vi "Set_Control_State.vi"(8 "Status/Errors in":refnum<vi>, 9 "Control Parameters [] in":T15[](array[typedef]) {"Aux Byte Value" format="%02x"; "Max Real Value" format="%#_6e"; "Min Real Value" format="%#_6e"; "dReal/dByte" format="%#_6e"; "Byte Value" format="%02x"; "Identifier" format="%02x"}, 10 "Main parameters in":T1={"Mode"={"Mode"=enum."Dialog", "Expert?"=FALSE, "Dialog?"=FALSE}, "Stop loop"={"Settings changed?"=FALSE, "Stop?"=refnum}, "Send message"={"Send mode"=enum."Get parameters", "Set parameter list"=0, "Get parameter list"=0, "Reset device"=0, "Length set settings message"=0, "Reset buttons?"=FALSE, "Reset Master?"=enum."General"}, "Write settings"={"Options"=enum."File 1"}, "Settings state"={"MAS locked?"=refnum, "SLV locked?"=refnum}, "Button refs"={"Stop program"=refnum, "Save settings"=refnum, "DAQ mode"=refnum, "Reset settings"=refnum, "Apply settings"=refnum, "Reset MAS"=refnum, "Reset SLV"=refnum, "Local DBase?"=refnum, "Last value DBase"=FALSE, "Database"=refnum, "Calibration"=refnum, "Save settings 2"=refnum}, "Update screen"={"Detector number"=0, "Hardware"=enum."None"}, "Files"={"Path config file"=path "", "Path def. ini file"=path "", "Path ini file 1"=path "", "Path ini file 2"=path "", "Path RBF file"=path ""}, "DB connection"={"connection reference"=refnum, "Connected?"=refnum, "ODBC Name"=""}, "Status_id"=refnum, "Time difference"=refnum, "Satellites"=refnum, "Alignment parameters"=refnum, "Page Statistics 2"=refnum, "Database"=refnum, "Page Statistics"=refnum} {"Update screen"."Detector number" format="%#.0f"; "Send message"."Reset device" format="%x"; "Send message"."Get parameter list" format="%x"; "Send message"."Set parameter list" format="%x"}) -> (0 "Status/Errors out":refnum<vi>, 1 "Control Parameters [] out":T15[](array[typedef]) {"Aux Byte Value" format="%02x"; "Max Real Value" format="%#_6e"; "Min Real Value" format="%#_6e"; "dReal/dByte" format="%#_6e"; "Byte Value" format="%02x"; "Identifier" format="%02x"}, 2 "Main parameters out":T1={"Mode"={"Mode"=enum."Dialog", "Expert?"=FALSE, "Dialog?"=FALSE}, "Stop loop"={"Settings changed?"=FALSE, "Stop?"=refnum}, "Send message"={"Send mode"=enum."Get parameters", "Set parameter list"=0, "Get parameter list"=0, "Reset device"=0, "Length set settings message"=0, "Reset buttons?"=FALSE, "Reset Master?"=enum."General"}, "Write settings"={"Options"=enum."File 1"}, "Settings state"={"MAS locked?"=refnum, "SLV locked?"=refnum}, "Button refs"={"Stop program"=refnum, "Save settings"=refnum, "DAQ mode"=refnum, "Reset settings"=refnum, "Apply settings"=refnum, "Reset MAS"=refnum, "Reset SLV"=refnum, "Local DBase?"=refnum, "Last value DBase"=FALSE, "Database"=refnum, "Calibration"=refnum, "Save settings 2"=refnum}, "Update screen"={"Detector number"=0, "Hardware"=enum."None"}, "Files"={"Path config file"=path "", "Path def. ini file"=path "", "Path ini file 1"=path "", "Path ini file 2"=path "", "Path RBF file"=path ""}, "DB connection"={"connection reference"=refnum, "Connected?"=refnum, "ODBC Name"=""}, "Status_id"=refnum, "Time difference"=refnum, "Satellites"=refnum, "Alignment parameters"=refnum, "Page Statistics 2"=refnum, "Database"=refnum, "Page Statistics"=refnum} {"Update screen"."Detector number" format="%#.0f"; "Send message"."Reset device" format="%x"; "Send message"."Get parameter list" format="%x"; "Send message"."Set parameter list" format="%x"})   [LabVIEW 2013]
uses:
  Controls/Control_Parameters.ctl
  Controls/Master.ctl
  Controls/Main_Parameters.ctl
  Controls/Mode.ctl
  Controls/Stop_Loop.ctl
  Controls/Send_Message.ctl
  Controls/Send_Message_Mode.ctl
  Controls/Write_Settings.ctl
  Controls/Write_Settings_Options.ctl
  Controls/Settings_State.ctl
  Controls/Button_Refs.ctl
  Controls/Update_Screen.ctl
  Controls/Files.ctl
  Controls/DB_Connection.ctl
  database/Connection.llb/Conn ObjectReference.ctl
  Controls/Get_Set_Buttons_mode.ctl
  Controls/TabPage_Events.ctl
  Controls/TabPage_Statistics.ctl
  Controls/Page_Thresholds.ctl
  Controls/Get_Set_Statistics_Options.ctl
  Controls/TabPage_Statistics2.ctl
  Controls/Tabpage_Satellites.ctl
panel:
  out "Last trigger Stack":u64[](array[numeric])
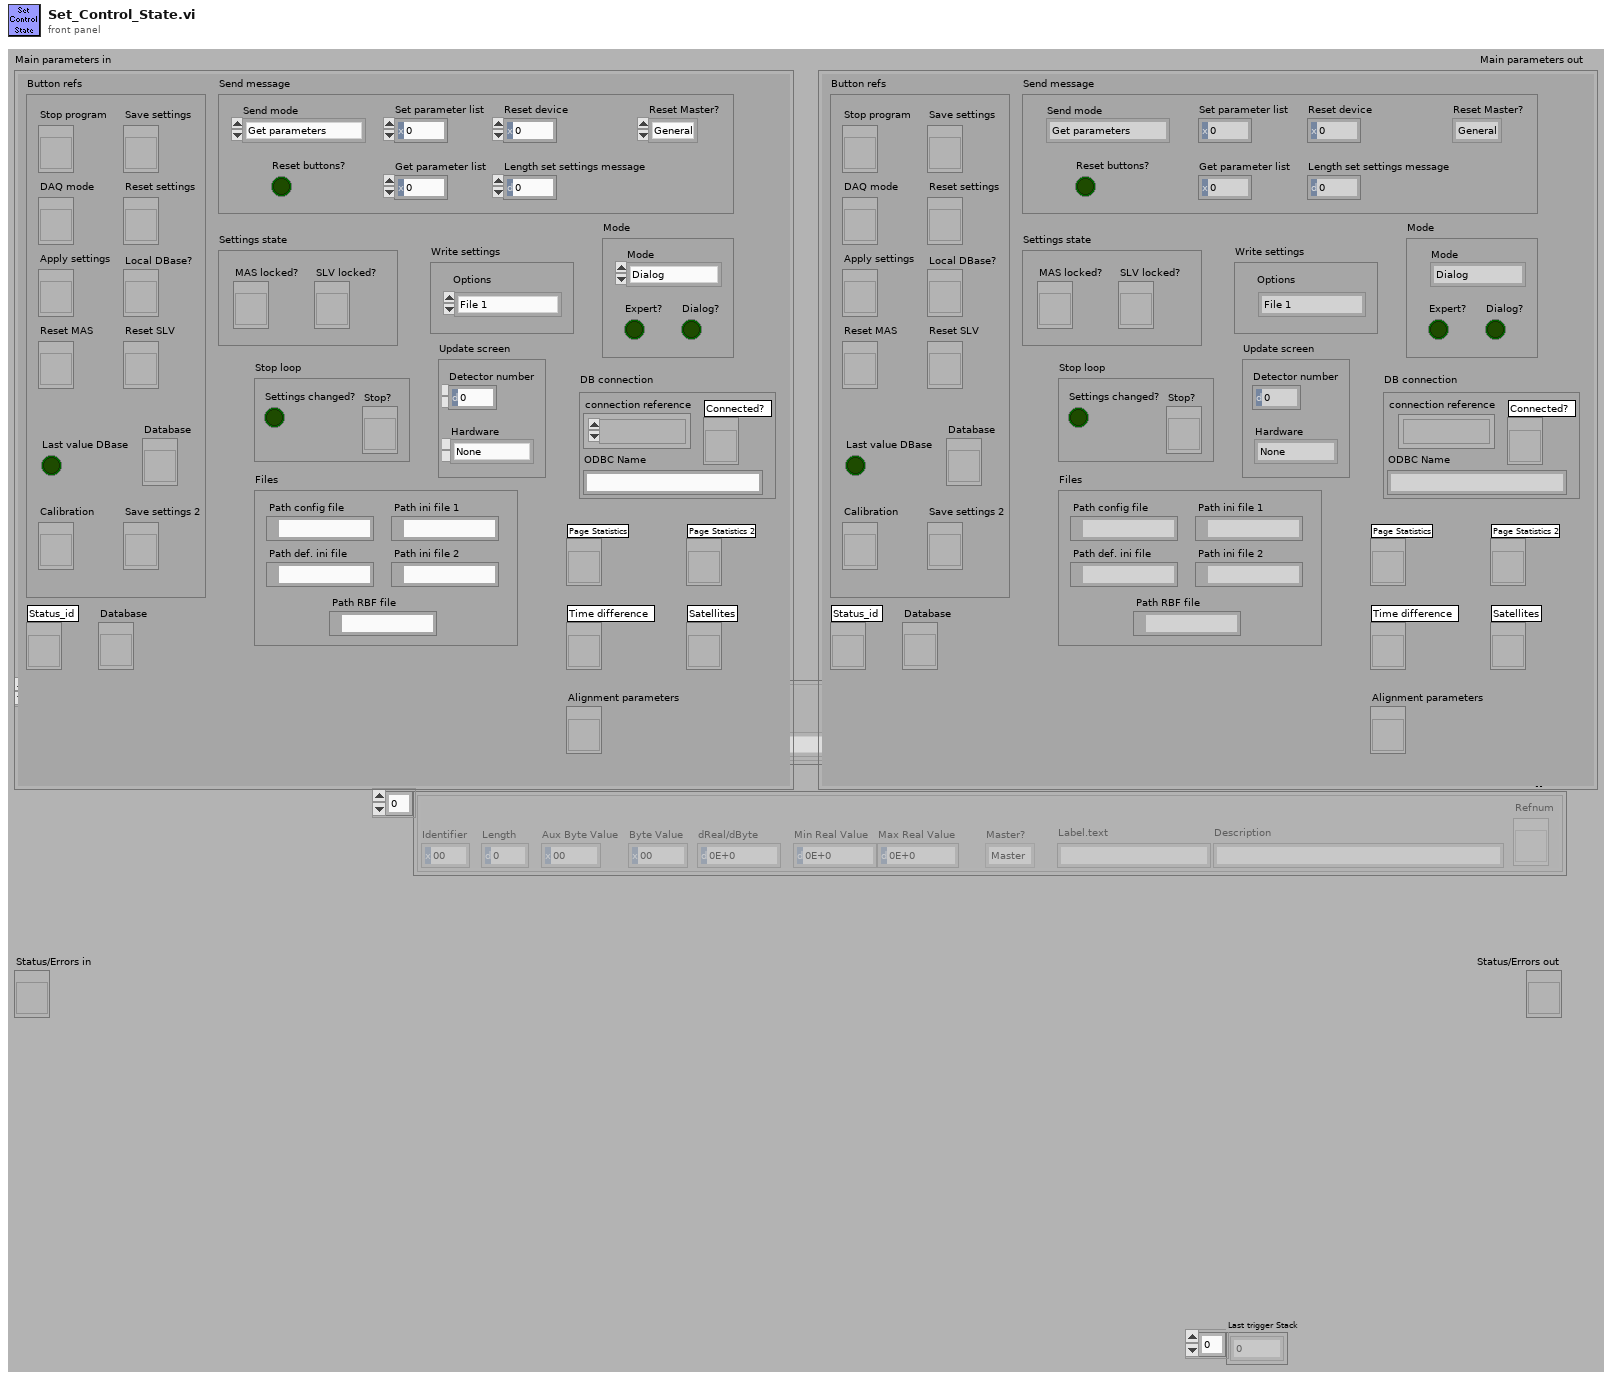
[diagram p1: front panel]
types:
  T1 = typedef "Main_Parameters.ctl" = cluster{"Mode":T2, "Stop loop":T3, "Send message":T4, "Write settings":T7, "Settings state":T9, "Button refs":T10, "Update screen":T11, "Files":T12, "DB connection":T13, "Status_id":refnum<vi>, "Time difference":refnum<vi>, "Satellites":refnum<vi>, "Alignment parameters":refnum<vi>, "Page Statistics 2":refnum<vi>, "Database":refnum<vi>, "Page Statistics":refnum<vi>}
  T2 = typedef "Mode.ctl" = cluster{"Mode":enum8{"Stop", "Dialog", "Hisparc II", "Hisparc II DAQ", "Alignment"}, "Expert?":bool, "Dialog?":bool}
  T3 = typedef "Stop_Loop.ctl" = cluster{"Settings changed?":bool, "Stop?":refnum<vi>}
  T4 = typedef "Send_Message.ctl" = cluster{"Send mode":T5, "Set parameter list":u8, "Get parameter list":u8, "Reset device":u8, "Length set settings message":i32, "Reset buttons?":bool, "Reset Master?":T6}
  T5 = typedef "Send_Message_Mode.ctl" = enum16{"Get parameters", "Set parameters", "From front panel", "From parameters", "Reset device", "Alignment"}
  T6 = typedef "Master.ctl" = enum16{"Master", "Slave", "General"}
  T7 = typedef "Write_Settings.ctl" = cluster{"Options":T8}
  T8 = typedef "Write_Settings_Options.ctl" = enum16{"File 1", "File 2", "Alignment", "Reset"}
  T9 = typedef "Settings_State.ctl" = cluster{"MAS locked?":refnum<vi>, "SLV locked?":refnum<vi>}
  T10 = typedef "Button_Refs.ctl" = cluster{"Stop program":refnum<vi>, "Save settings":refnum<vi>, "DAQ mode":refnum<vi>, "Reset settings":refnum<vi>, "Apply settings":refnum<vi>, "Reset MAS":refnum<vi>, "Reset SLV":refnum<vi>, "Local DBase?":refnum<vi>, "Last value DBase":bool, "Database":refnum<vi>, "Calibration":refnum<vi>, "Save settings 2":refnum<vi>}
  T11 = typedef "Update_Screen.ctl" = cluster{"Detector number":u16, "Hardware":enum8{"None", "HiSPARC I", "HiSPARC II", "HiSPARC III", "Unknown"}}
  T12 = typedef "Files.ctl" = cluster{"Path config file":path, "Path def. ini file":path, "Path ini file 1":path, "Path ini file 2":path, "Path RBF file":path}
  T13 = typedef "DB_Connection.ctl" = cluster{"connection reference":T14, "Connected?":refnum<vi>, "ODBC Name":string}
  T14 = typedef "Conn ObjectReference.ctl" = refnum<k1>
  T15 = typedef "Control_Parameters.ctl" = cluster{"Identifier":u8, "Length":u16, "Byte Value":u32, "dReal/dByte":dbl, "Min Real Value":dbl, "Max Real Value":dbl, "Master?":T6, "Label.text":string, "Description":string, "Refnum":refnum<vi>, "Aux Byte Value":u32}
  T16 = typedef "Tabpage_Satellites.ctl" = cluster{"Satellites_online":dbl[], "Satellite_signal":dbl[][], "Total_signal_strength":dbl[], "First time?":bool}
  T17 = typedef "TabPage_Statistics2.ctl" = cluster{"Baseline_overshoot":dbl, "St.Dev.overshoot":dbl, "Data points overshoot":dbl, "Time difference overshoot":dbl, "Time_difference_zoom_count":dbl, "Baseline.His":cluster{"t0":i32, "dt":i32, "Histogram":i32[][]}, "St._dev.His":cluster{"t0":i32, "dt":i32, "Histogram":i32[][]}, "Trace_length.His":cluster{"t0":i32, "dt":i32, "Histogram":i32[][]}, "Time_difference.His_zoom":cluster{"t0":i32, "dt":i32, "Histogram":i32[][]}, "Time_difference.His":cluster{"t0":i32, "dt":i32, "Histogram":i32[][]}, "Baselin Entries":u64, "Baseline Overshoots":u64, "Time Entries ":u64, "Time  Overshoots ":u64, "St.dev. Entries ":u64, "St.dev.  Overshoots ":u64, "Length  Entries ":u64, "Length Overshoots ":u64, "Time zoom Entries ":u64, "Time zoom Overshoots ":u64}
  T18 = typedef "Get_Set_Statistics_Options.ctl" = enum16{"Get", "Set singles", "Set events"}
  T19 = typedef "TabPage_Statistics.ctl" = cluster{"Thresh_Count_MAS":T20, "Thresh_Count_SLV":T20, "Count":bool, "Time_to_count":u32, "Time":u32, "Time_to_count_ref":refnum<vi>, "Counting?":bool, "Baseline_MAS_Ch1":i16, "Baseline_MAS_Ch2":i16, "Baseline_SLV_Ch1":i16, "Baseline_SLV_Ch2":i16, "Basel_Err_MAS_Ch1":u32, "Basel_Err_MAS_Ch2":u32, "Basel_Err_SLV_Ch1":u32, "Basel_Err_SLV_Ch2":u32, "Peaks_Overshoot":dbl, "Height_Overshoot":dbl, "Integrals_Overshoot":dbl, "Last_event":dbl, "Total_Trigger":u32, "Av_Trigger":dbl, "Number of peaks":cluster{"t0":i32, "dt":i32, "Histogram":i32[][]}, "Pulse height":cluster{"t0":i32, "dt":i32, "Histogram":i32[][]}, "Integral":cluster{"t0":i32, "dt":i32, "Histogram":i32[][]}, "Number of peaks Entries":u64, "Number of peaks Overshoots":u64, "Pulse height  Entries":u64, "Pulse height Overshoots":u64, "Integral Entries":u64, "Integral Overshoots":u64, "Last trigger Stack":refnum<vi>}
  T20 = typedef "Page_Thresholds.ctl" = cluster{"Sing_Ch1_low":u32, "Sing_Ch1_high":u32, "Sing_Ch2_low":u32, "Sing_Ch2_high":u32, "Total_Ch1_low":u32, "Total_Ch1_high":u32, "Total_Ch2_low":u32, "Total_Ch2_high":u32, "Av_Ch1_low":dbl, "Av_Ch1_high":dbl, "Av_Ch2_low":dbl, "Av_Ch2_high":dbl}
  T21 = typedef "TabPage_Events.ctl" = cluster{"Det_Numb":u16, "GPS_Timestamp":string, "Trigger_Pattern":cluster{"Master ch. 1 lower threshold":bool, "Master ch. 1 higher threshold":bool, "Master ch. 2 lower threshold":bool, "Master ch. 2 higher threshold":bool, "Slave ch. 1 lower threshold":bool, "Slave ch. 1 higher threshold":bool, "Slave ch. 2 lower threshold":bool, "Slave ch. 2 higher threshold":bool, "External trigger":bool, "Slave present?":bool, "Ch. 1 low comparator master":bool, "Ch. 1 high comparator master":bool, "Ch. 2 low comparator master":bool, "Ch. 2 high comparator master":bool, "Ch. 1 low comparator slave":bool, "Ch. 1 high comparator slave":bool, "Ch. 2 low comparator slave":bool, "Ch. 2 high comparator slave":bool}, "Traces":dbl[][], "MAS_Status_Events":bool, "MAS_Vers_Numb":string, "SLV_Status_Events":bool, "SLV_Vers_Numb":string, "DBase_connected?":bool, "MAS_GPS_Long":dbl, "MAS_GPS_Lat":dbl, "MAS_GPS_Alt":dbl, "Hardware":enum8{"None", "HiSPARC I", "HiSPARC II", "HiSPARC III", "Unknown"}}
  T22 = typedef "Get_Set_Buttons_mode.ctl" = enum16{"Get", "Get DAQ", "Set", "Set settings"}
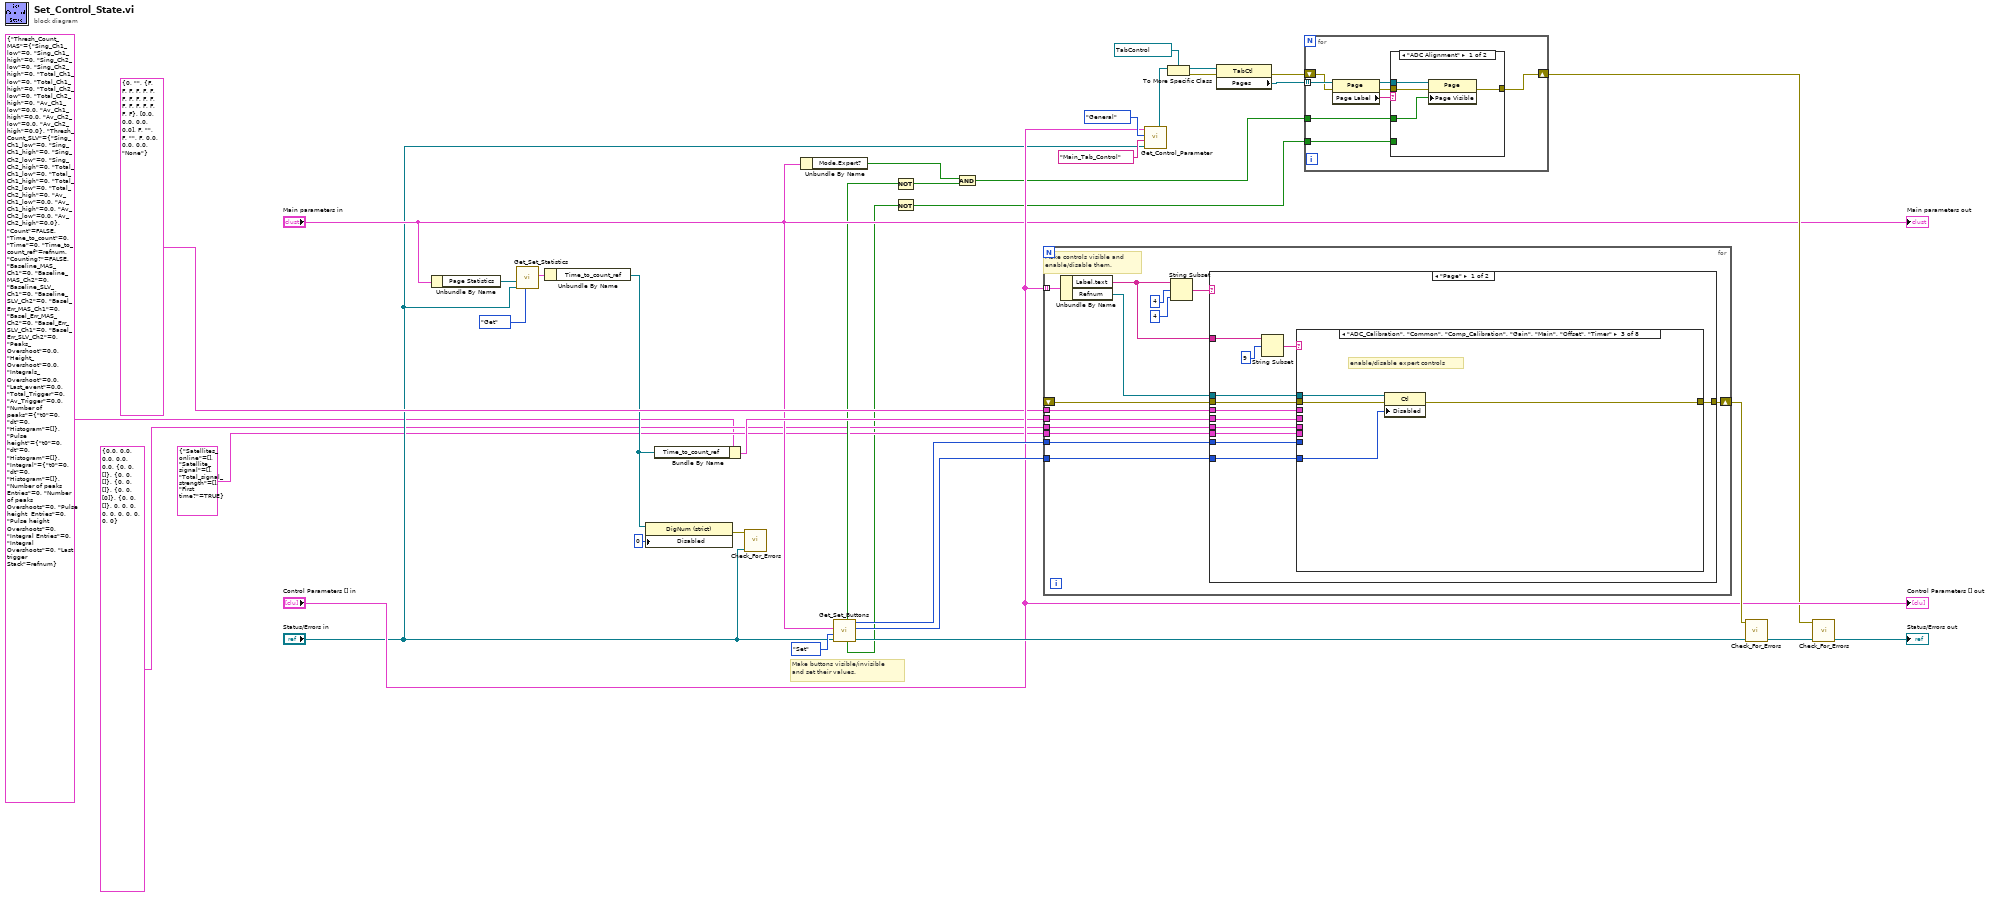
[diagram p0: block diagram]
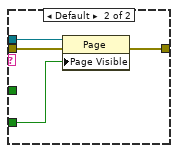
[diagram p2: hidden frame]
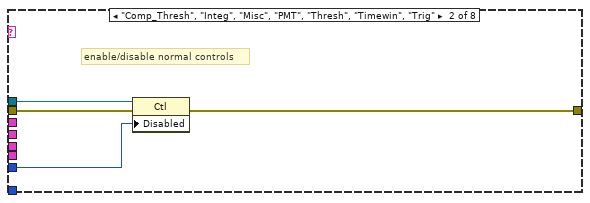
[diagram p4: hidden frame]
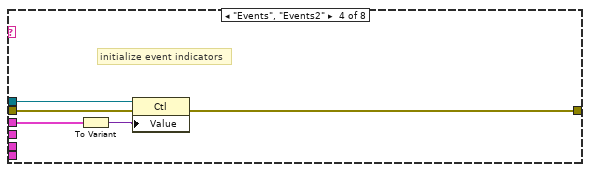
[diagram p5: hidden frame]
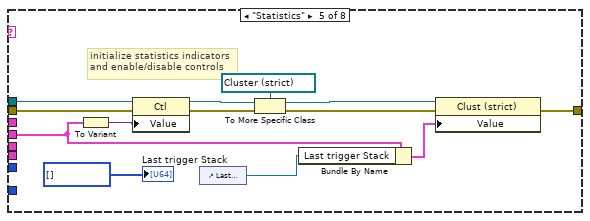
[diagram p6: hidden frame]
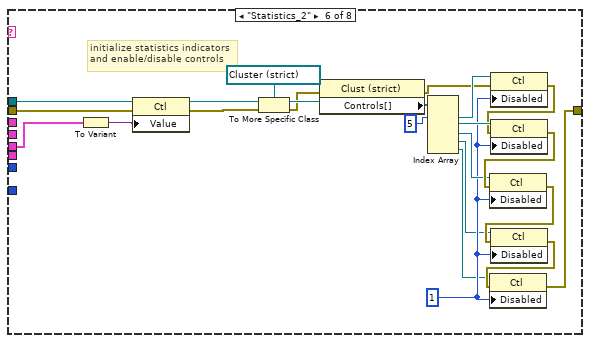
[diagram p7: hidden frame]
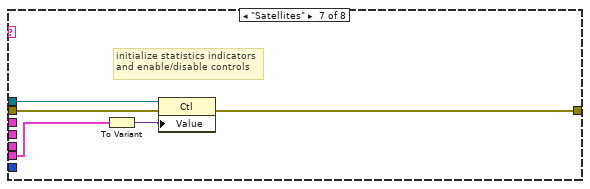
[diagram p8: hidden frame]
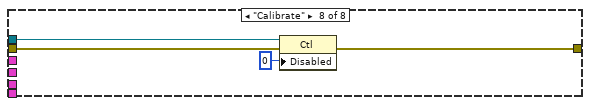
[diagram p9: hidden frame]
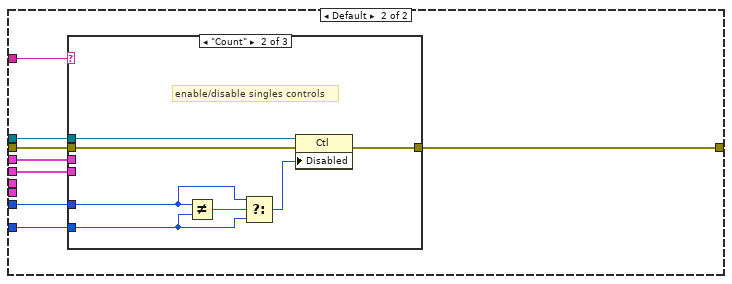
[diagram p10: hidden frame]
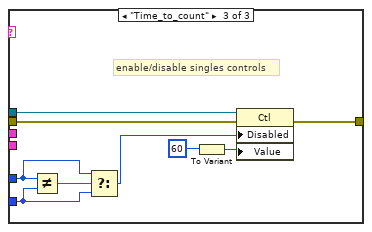
[diagram p12: hidden frame]
diagram:
  # "Make buttons visible/invisible\nand set their values."
  # "Make controls visible and\nenable/disable them."
  n1 = Unbundle By Name("Main parameters in") -> ("Page Statistics"=w1:refnum<vi>)
  n2 = call "Get_Set_Statistics.vi"("Page Statistics in"=w1, "Status/Errors in"="Status/Errors in", "Get/Set"=Get_Set_Statistics_Options."Get") -> ("Value out"=w16:T19)  [unwired: 2 in, 5 out]
  n3 = Unbundle By Name(w16) -> ("Time_to_count_ref"=w7:refnum<vi>)
  n4 = property class="DigNum (strict)"(reference=w7, "Disabled"=u8 0) -> (error out=w9:errorcluster)  [unwired: 1 in, 1 out]
  n5 = Bundle By Name(cluster=T19 {"Thresh_Count_MAS"={"Sing_Ch1_low"=0, "Sing_Ch1_high"=0, "Sing_Ch2_low"=0, "Sing_Ch2_high"=0, "Total_Ch1_low"=0, "Total_Ch1_high"=0, "Total_Ch2_low"=0, "Total_Ch2_high"=0, "Av_Ch1_low"=0.0, "Av_Ch1_high"=0.0, "Av_Ch2_low"=0.0, "Av_Ch2_high"=0.0}, "Thresh_Count_SLV"={"Sing_Ch1_low"=0, "Sing_Ch1_high"=0, "Sing_Ch2_low"=0, "Sing_Ch2_high"=0, "Total_Ch1_low"=0, "Total_Ch1_high"=0, "Total_Ch2_low"=0, "Total_Ch2_high"=0, "Av_Ch1_low"=0.0, "Av_Ch1_high"=0.0, "Av_Ch2_low"=0.0, "Av_Ch2_high"=0.0}, "Count"=FALSE, "Time_to_count"=0, "Time"=0, "Time_to_count_ref"=refnum, "Counting?"=FALSE, "Baseline_MAS_Ch1"=0, "Baseline_MAS_Ch2"=0, "Baseline_SLV_Ch1"=0, "Baseline_SLV_Ch2"=0, "Basel_Err_MAS_Ch1"=0, "Basel_Err_MAS_Ch2"=0, "Basel_Err_SLV_Ch1"=0, "Basel_Err_SLV_Ch2"=0, "Peaks_Overshoot"=0.0, "Height_Overshoot"=0.0, "Integrals_Overshoot"=0.0, "Last_event"=0.0, "Total_Trigger"=0, "Av_Trigger"=0.0, "Number of peaks"={"t0"=0, "dt"=0, "Histogram"=[]}, "Pulse height"={"t0"=0, "dt"=0, "Histogram"=[]}, "Integral"={"t0"=0, "dt"=0, "Histogram"=[]}, "Number of peaks Entries"=0, "Number of peaks Overshoots"=0, "Pulse height  Entries"=0, "Pulse height Overshoots"=0, "Integral Entries"=0, "Integral Overshoots"=0, "Last trigger Stack"=refnum} ("GEN_Page_Statistics"), "Time_to_count_ref"=w7) -> (w15:T19)
  n6 = call "Check_For_Errors.vi"("Status/Errors in"="Status/Errors in", "error in"=w9) -> ()  [unwired: 10 out]
  n7 = Unbundle By Name("Main parameters in") -> ("Mode.Expert?"=w11:bool)
  n8 = call "Get_Set_Buttons.vi"("Status/Errors in"="Status/Errors in", "Set?"=Get_Set_Buttons_mode."Set", "Main parameters"="Main parameters in") -> ("Status/Errors out"=w32:refnum<vi>, "Enabled State Expert"=w33:u8, "Enabled State Normal"=w34:u8, "Calibration value"=w2:bool, "DAQ mode value"=w13:bool)  [unwired: 1 in, 3 out]
  n9 = Not(x=w13) -> (.not. x?=w12:bool)
  n10 = Not(x=w2) -> (.not. x?=w19:bool)
  n11 = And(x=w11, y=w12) -> (x .and. y?=w10:bool)
  n12 = for {
    tunnel: "Control Parameters [] in" -> [w47] mode=indexing
    tunnel: w34 -> [w45]
    shift-right: [w43] -> w36
    shift-left: _ -> [w44]
    tunnel: w33 -> [w42]
    tunnel: T21 {"Det_Numb"=0, "GPS_Timestamp"="", "Trigger_Pattern"={"Master ch. 1 lower threshold"=FALSE, "Master ch. 1 higher threshold"=FALSE, "Master ch. 2 lower threshold"=FALSE, "Master ch. 2 higher threshold"=FALSE, "Slave ch. 1 lower threshold"=FALSE, "Slave ch. 1 higher threshold"=FALSE, "Slave ch. 2 lower threshold"=FALSE, "Slave ch. 2 higher threshold"=FALSE, "External trigger"=FALSE, "Slave present?"=FALSE, "Ch. 1 low comparator master"=FALSE, "Ch. 1 high comparator master"=FALSE, "Ch. 2 low comparator master"=FALSE, "Ch. 2 high comparator master"=FALSE, "Ch. 1 low comparator slave"=FALSE, "Ch. 1 high comparator slave"=FALSE, "Ch. 2 low comparator slave"=FALSE, "Ch. 2 high comparator slave"=FALSE}, "Traces"=[[0.0, 0.0], [0.0, 0.0]], "MAS_Status_Events"=FALSE, "MAS_Vers_Numb"="", "SLV_Status_Events"=FALSE, "SLV_Vers_Numb"="", "DBase_connected?"=FALSE, "MAS_GPS_Long"=0.0, "MAS_GPS_Lat"=0.0, "MAS_GPS_Alt"=0.0, "Hardware"=enum."None"} ("Events") -> [w40]
    tunnel: w15 -> [w39]
    tunnel: T17 {"Baseline_overshoot"=0.0, "St.Dev.overshoot"=0.0, "Data points overshoot"=0.0, "Time difference overshoot"=0.0, "Time_difference_zoom_count"=0.0, "Baseline.His"={"t0"=0, "dt"=0, "Histogram"=[]}, "St._dev.His"={"t0"=0, "dt"=0, "Histogram"=[]}, "Trace_length.His"={"t0"=0, "dt"=0, "Histogram"=[]}, "Time_difference.His_zoom"={"t0"=0, "dt"=0, "Histogram"=[[0]]}, "Time_difference.His"={"t0"=0, "dt"=0, "Histogram"=[]}, "Baselin Entries"=0, "Baseline Overshoots"=0, "Time Entries "=0, "Time  Overshoots "=0, "St.dev. Entries "=0, "St.dev.  Overshoots "=0, "Length  Entries "=0, "Length Overshoots "=0, "Time zoom Entries "=0, "Time zoom Overshoots "=0} ("GEN_Page_Statistics_2") -> [w38]
    tunnel: T16 {"Satellites_online"=[], "Satellite_signal"=[], "Total_signal_strength"=[], "First time?"=TRUE} ("GEN_Page_Statistics_2") -> [w37]
    n13 = Unbundle By Name(w47) -> ("Label.text"=w46:string, "Refnum"=w41:refnum<vi>)
    n14 = String Subset(string=w46, offset (0)=4, length (rest)=4 ("length (rest)")) -> (substring=w49:string)
    n15 = case shown="\"Page\"" w49 {
      tunnel: w41 -> [w56 w126]
      tunnel: w46 -> [w60 w122]
      tunnel: w45 -> [w59 w129]
      tunnel: w44 -> [w55 w125]
      tunnel: [w58 w128] -> w43
      tunnel: w42 -> [w57 w127]
      tunnel: w40 -> [w54 w124]
      tunnel: w39 -> [w53 w123]
      tunnel: w38 -> [w52 _]
      tunnel: w37 -> [w51 _]
      frame "Page" {
        n16 = String Subset(string=w60, offset (0)=9) -> (substring=w61:string)  [unwired: 1 out]
        n17 = case shown="\"ADC_Calibration\", \"Common\", \"Comp_Calibration\", \"Gain\", \"Main\", \"Offset\", \"Timer\"" w61 {
          tunnel: w56 -> [_ w67 w71 w76 w89 w108 w116 w120]
          tunnel: w59 -> [_ w66 _ _ _ _ _ _]
          tunnel: w55 -> [w63 w65 w70 w75 w88 w112 w115 w119]
          tunnel: [w63 w64 w69 w74 w82 w90 w113 w121] -> w58
          tunnel: w57 -> [_ _ w68 _ _ _ _ _]
          tunnel: w54 -> [_ _ _ w72 _ _ _ _]
          tunnel: w53 -> [_ _ _ _ w79 _ _ _]
          tunnel: w52 -> [_ _ _ _ _ w110 _ _]
          tunnel: w51 -> [_ _ _ _ _ _ w114 _]
          frame Default {
          }
          frame "Comp_Thresh", "Integ", "Misc", "PMT", "Thresh", "Timewin", "Trig" {
            # "enable/disable normal controls"
            n18 = property class="Ctl"(reference=w67, error in=w65, "Disabled"=w66) -> (error out=w64:errorcluster)  [unwired: 1 out]
          }
          frame "ADC_Calibration", "Common", "Comp_Calibration", "Gain", "Main", "Offset", "Timer" {
            # "enable/disable expert controls"
            n19 = property class="Ctl"(reference=w71, error in=w70, "Disabled"=w68) -> (error out=w69:errorcluster)  [unwired: 1 out]
          }
          frame "Events", "Events2" {
            # "initialize event indicators"
            n20 = To Variant(anything=w72) -> (Variant=w73:variant)
            n21 = property class="Ctl"(reference=w76, error in=w75, "Value"=w73) -> (error out=w74:errorcluster)  [unwired: 1 out]
          }
          frame "Statistics" {
            # "initialize statistics indicators\nand enable/disable controls"
            n22 = To Variant(anything=w79) -> (Variant=w87:variant)
            n23 = property class="Ctl"(reference=w89, error in=w88, "Value"=w87) -> (reference out=w84:refnum<vi>, error out=w83:errorcluster)
            n24 = control-ref of="Last trigger Stack"() -> (w81:refnum<vi>)
            n25 = To More Specific Class(target class=refnum<vi> refnum ("GEN_Page_Statistics"), reference=w84, error in=w83) -> (specific class reference=w86:refnum<vi>, error out=w85:errorcluster)
            n26 = Bundle By Name(cluster=w79, "Last trigger Stack"=w81) -> (w78:T19)
            n27 = property class="Clust (strict)"(reference=w86, error in=w85, "Value"=w78) -> (error out=w82:errorcluster)  [unwired: 1 out]
            "Last trigger Stack" <- u64[] [] ("Last trigger Stack")
          }
          frame "Statistics_2" {
            w93 = u8 1 ("index")
            # "initialize statistics indicators\nand enable/disable controls"
            n28 = To Variant(anything=w110) -> (Variant=w111:variant)
            n29 = property class="Ctl"(reference=w108, error in=w112, "Value"=w111) -> (reference out=w103:refnum<vi>, error out=w104:errorcluster)
            n30 = To More Specific Class(target class=refnum<vi> refnum ("GEN_Page_Statistics_2"), reference=w103, error in=w104) -> (specific class reference=w107:refnum<vi>, error out=w100:errorcluster)
            n31 = property class="Clust (strict)"(reference=w107, error in=w100) -> (error out=w99:errorcluster, "Controls[]"=w106:refnum<vi>[])  [unwired: 1 out]
            n32 = Index Array(array=w106, index #1=5 ("index")) -> (element #1=w102:refnum<vi>, element #2=w101:refnum<vi>, element #3=w96:refnum<vi>, element #4=w92:refnum<vi>, element #5=w91:refnum<vi>)  [unwired: 4 in]
            n33 = property class="Ctl"(reference=w102, error in=w99, "Disabled"=w93) -> (error out=w98:errorcluster)  [unwired: 1 out]
            n34 = property class="Ctl"(reference=w101, error in=w98, "Disabled"=w93) -> (error out=w97:errorcluster)  [unwired: 1 out]
            n35 = property class="Ctl"(reference=w96, error in=w97, "Disabled"=w93) -> (error out=w95:errorcluster)  [unwired: 1 out]
            n36 = property class="Ctl"(reference=w92, error in=w95, "Disabled"=w93) -> (error out=w94:errorcluster)  [unwired: 1 out]
            n37 = property class="Ctl"(reference=w91, error in=w94, "Disabled"=w93) -> (error out=w90:errorcluster)  [unwired: 1 out]
          }
          frame "Satellites" {
            # "initialize statistics indicators\nand enable/disable controls"
            n38 = To Variant(anything=w114) -> (Variant=w117:variant)
            n39 = property class="Ctl"(reference=w116, error in=w115, "Value"=w117) -> (error out=w113:errorcluster)  [unwired: 1 out]
          }
          frame "Calibrate" {
            n40 = property class="Ctl"(reference=w120, error in=w119, "Disabled"=u8 0) -> (error out=w121:errorcluster)  [unwired: 1 out]
          }
        }
      }
      frame Default {
        n41 = case shown="\"Count\"" w122 {
          tunnel: w126 -> [_ w137 w146]
          tunnel: w129 -> [_ w132 w141]
          tunnel: w125 -> [w130 w136 w145]
          tunnel: [w130 w135 w144] -> w128
          tunnel: w127 -> [_ w131 w140]
          tunnel: w124 -> [_ _ _]
          tunnel: w123 -> [_ _ _]
          frame Default {
          }
          frame "Count" {
            # "enable/disable singles controls"
            n42 = Not Equal?(x=w132, y=w131) -> (x != y?=w133:bool)
            n43 = Select(t=w132, s=w133, f=w131) -> (s? t:f=w134:u8)
            n44 = property class="Ctl"(reference=w137, error in=w136, "Disabled"=w134) -> (error out=w135:errorcluster)  [unwired: 1 out]
          }
          frame "Time_to_count" {
            # "enable/disable singles controls"
            n45 = Not Equal?(x=w141, y=w140) -> (x != y?=w142:bool)
            n46 = Select(t=w141, s=w142, f=w140) -> (s? t:f=w143:u8)
            n47 = To Variant(anything=60) -> (Variant=w139:variant)
            n48 = property class="Ctl"(reference=w146, error in=w145, "Disabled"=w143, "Value"=w139) -> (error out=w144:errorcluster)  [unwired: 1 out]
          }
        }
      }
    }
  }
  n49 = call "Get_Control_Parameter.vi"("Status/Errors in"="Status/Errors in", "Label.text in"="Main_Tab_Control", "Master?"=Master."General", "Control Parameters [] in"="Control Parameters [] in") -> ("Refnum"=w26:refnum<vi>)  [unwired: 7 out]
  n50 = To More Specific Class(target class=refnum<vi> refnum ("Main Tab Control in"), reference=w26) -> (specific class reference=w24:refnum<vi>, error out=w25:errorcluster)  [unwired: 1 in]
  n51 = property class="TabCtl"(reference=w24, error in=w25) -> (error out=w30:errorcluster, "Pages"=w31:refnum<vi>[])  [unwired: 1 out]
  n52 = for {
    tunnel: w31 -> [w154] mode=indexing
    shift-right: [w149] -> w22
    shift-left: w30 -> [w151]
    tunnel: w10 -> [w148]
    tunnel: w19 -> [w147]
    n53 = property class="Page"(reference=w154, error in=w151) -> (reference out=w152:refnum<vi>, error out=w150:errorcluster, "Page Label"=w153:string)
    n54 = case shown="\"ADC Alignment\"" w153 {
      tunnel: w152 -> [w158 w162]
      tunnel: w150 -> [w157 w161]
      tunnel: [w156 w160] -> w149
      tunnel: w148 -> [w155 _]
      tunnel: w147 -> [_ w159]
      frame "ADC Alignment" {
        n55 = property class="Page"(reference=w158, error in=w157, "Page Visible"=w155) -> (error out=w156:errorcluster)  [unwired: 1 out]
      }
      frame Default {
        n56 = property class="Page"(reference=w162, error in=w161, "Page Visible"=w159) -> (error out=w160:errorcluster)  [unwired: 1 out]
      }
    }
  }
  n57 = call "Check_For_Errors.vi"("Status/Errors in"=w32, "error in"=w36) -> ("Status/Errors out"=w21:refnum<vi>)  [unwired: 9 out]
  n58 = call "Check_For_Errors.vi"("Status/Errors in"=w21, "error in"=w22) -> ("Status/Errors out"=→"Status/Errors out":refnum<vi>)  [unwired: 9 out]
  "Control Parameters [] out" <- "Control Parameters [] in"
  "Main parameters out" <- "Main parameters in"
